vi "subSave_XYTfilename.vi"(4 "Xi":i32, 5 "Tiling?":bool, 6 "Yi":i32, 11 "Z-stack cluster in":T1={"Timelapse Acquired"=1, "File path"=path "C:/Users/ZouOptics/Desktop/TEST", "Z-Stack"={"Z end"=0.0, "Step Num"=1, "Step Size"=2.0, "Z0"=3471.0, "z-stack?"=FALSE}, "Frames to avg."=20, "Image Info Ref"=refnum, "Camera Ctrl"={"Chosen Camera"=0, "ROI selection"=0, "Live"=FALSE, "ROI define"=FALSE, "Snap"=FALSE, "ROI update"=FALSE, "ROI previous "=FALSE, "ROI"={"Bin"=2, "ROI"={"x offset"=256, "y offset"=256, "x width"=512, "y width"=512}}, "Exposure (ms)"=100.0, "Symmetrical"=FALSE, "Autoscale"=TRUE, "Scale"={"Scale.Min"=0, "Scale.Max"=6038}}} {"Camera Ctrl"."Scale"."Scale.Max" min=1 max=5000 step=1; "Camera Ctrl"."Scale"."Scale.Min" min=1 max=5000 step=1; "Camera Ctrl"."Exposure (ms)" min=1.0 max=5000.0 step=1.0; "Camera Ctrl"."ROI"."ROI"."x offset" min=1 max=512 step=1; "Camera Ctrl"."ROI"."ROI"."y offset" min=1 max=512 step=1; "Camera Ctrl"."ROI"."ROI"."x width" min=1 max=512 step=1; "Camera Ctrl"."ROI"."ROI"."y width" min=1 max=512 step=1; "Camera Ctrl"."ROI"."Bin" items=["1x1"=1, "2x2"=2, "4x4"=4]; "Camera Ctrl"."ROI selection" items=["Full ROI", "Central quad", "Confocal"]; "Camera Ctrl"."Chosen Camera" items=["Left", "Right"]}) -> (3 "Z-stack cluster out":T1={"Timelapse Acquired"=1, "File path"=path "C:/Users/ZouOptics/Desktop/TEST", "Z-Stack"={"Z end"=0.0, "Step Num"=1, "Step Size"=2.0, "Z0"=3471.0, "z-stack?"=FALSE}, "Frames to avg."=20, "Image Info Ref"=refnum, "Camera Ctrl"={"Chosen Camera"=0, "ROI selection"=0, "Live"=FALSE, "ROI define"=FALSE, "Snap"=FALSE, "ROI update"=FALSE, "ROI previous "=FALSE, "ROI"={"Bin"=2, "ROI"={"x offset"=256, "y offset"=256, "x width"=512, "y width"=512}}, "Exposure (ms)"=100.0, "Symmetrical"=FALSE, "Autoscale"=TRUE, "Scale"={"Scale.Min"=0, "Scale.Max"=6038}}} {"Camera Ctrl"."Scale"."Scale.Max" min=1 max=5000 step=1; "Camera Ctrl"."Scale"."Scale.Min" min=1 max=5000 step=1; "Camera Ctrl"."Exposure (ms)" min=1.0 max=5000.0 step=1.0; "Camera Ctrl"."ROI"."ROI"."x offset" min=1 max=512 step=1; "Camera Ctrl"."ROI"."ROI"."y offset" min=1 max=512 step=1; "Camera Ctrl"."ROI"."ROI"."x width" min=1 max=512 step=1; "Camera Ctrl"."ROI"."ROI"."y width" min=1 max=512 step=1; "Camera Ctrl"."ROI"."Bin" items=["1x1"=1, "2x2"=2, "4x4"=4]; "Camera Ctrl"."ROI selection" items=["Full ROI", "Central quad", "Confocal"]; "Camera Ctrl"."Chosen Camera" items=["Left", "Right"]})   [LabVIEW 2015]
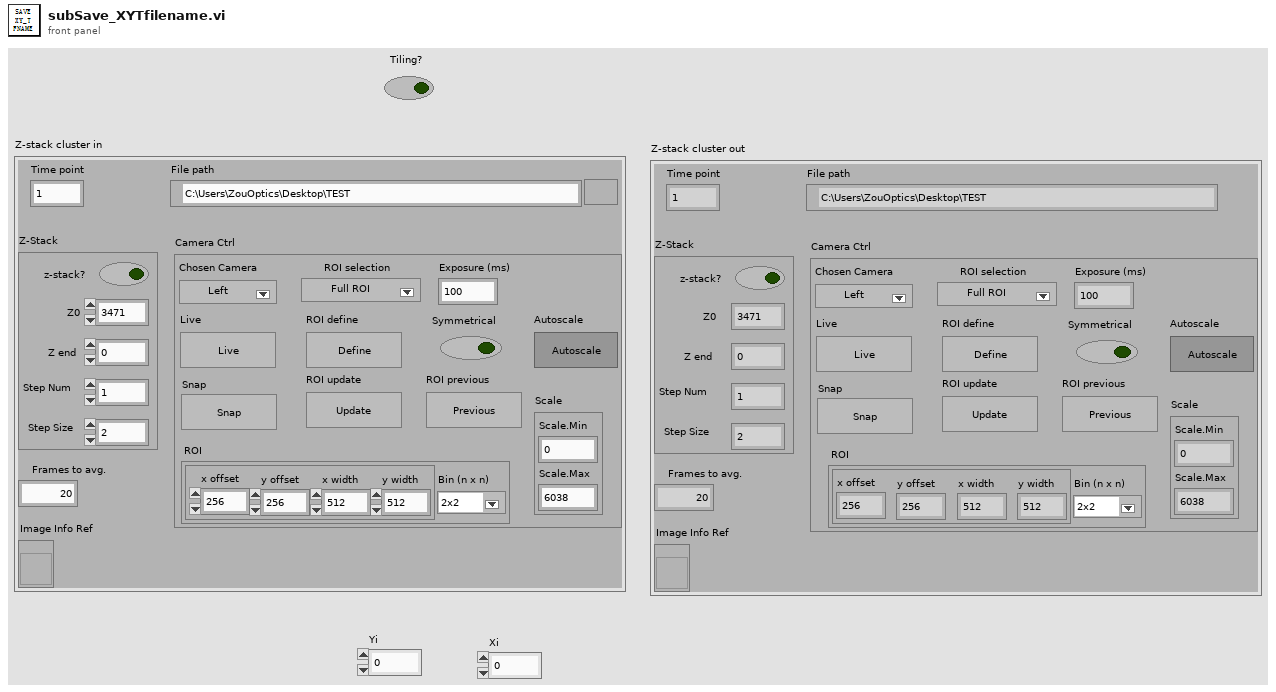
[diagram p1: front panel]
types:
  T1 = cluster{"Timelapse Acquired":i32, "File path":path, "Z-Stack":cluster{"Z end":dbl, "Step Num":i32, "Step Size":dbl, "Z0":dbl, "z-stack?":bool}, "Frames to avg.":i32, "Image Info Ref":refnum<vi>, "Camera Ctrl":cluster{"Chosen Camera":u32, "ROI selection":u16, "Live":bool, "ROI define":bool, "Snap":bool, "ROI update":bool, "ROI previous ":bool, "ROI":cluster{"Bin":u16, "ROI":cluster{"x offset":i32, "y offset":i32, "x width":i32, "y width":i32}}, "Exposure (ms)":dbl, "Symmetrical":bool, "Autoscale":bool, "Scale":cluster{"Scale.Min":i32, "Scale.Max":i32}}}
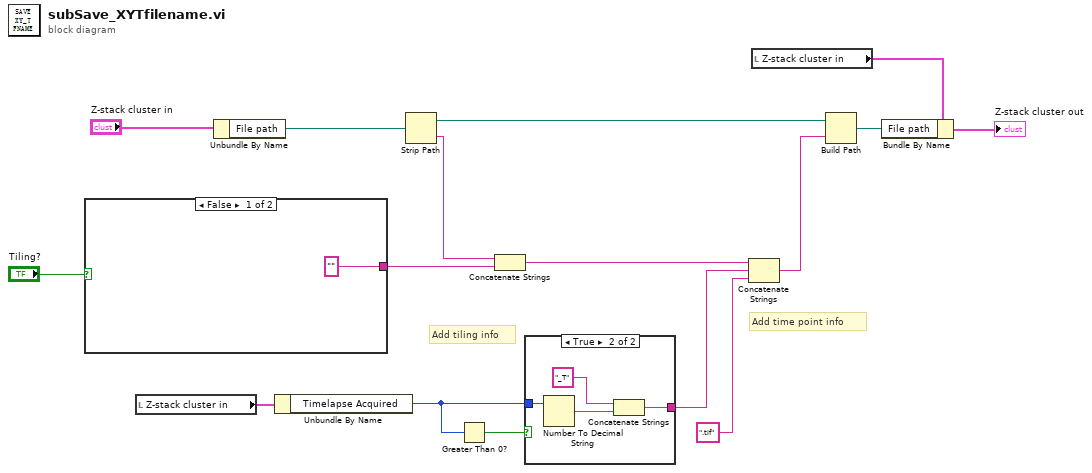
[diagram p0: block diagram]
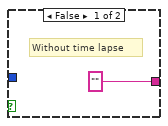
[diagram p2: hidden frame]
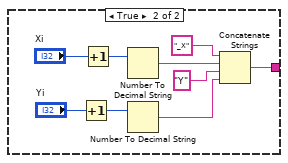
[diagram p3: hidden frame]
diagram:
  # "Add time point info"
  # "Add tiling info"
  n1 = case shown="False" "Tiling?" {
    tunnel: ["" w24] -> w10
    frame False {
    }
    frame True {
      n2 = Increment(x="Yi") -> (x+1=w25:i32)
      n3 = Increment(x="Xi") -> (x+1=w26:i32)
      n4 = Number To Decimal String(number=w26) -> (decimal integer string=w20:string)  [unwired: 1 in]
      n5 = Number To Decimal String(number=w25) -> (decimal integer string=w18:string)  [unwired: 1 in]
      n6 = Concatenate Strings("_X" ("string"), w20, "Y" ("string"), w18) -> (w24:string)
    }
  }
  n7 = local read "Z-stack cluster in"() -> (w13:T1)
  n8 = Unbundle By Name("Z-stack cluster in") -> ("File path"=w14:path)
  n9 = Unbundle By Name(w13) -> ("Timelapse Acquired"=w8:i32)
  n10 = Strip Path(path=w14) -> (stripped path=w16:path, name=w11:string)
  n11 = Greater Than 0?(x=w8) -> (x > 0?=w9:bool)
  n12 = Concatenate Strings(w11, w10) -> (w4:string)
  n13 = case shown="True" w9 {
    tunnel: w8 -> [_ w31]
    tunnel: ["" w28] -> w7
    frame False {
      # "Without time lapse"
    }
    frame True {
      n14 = Number To Decimal String(number=w31) -> (decimal integer string=w29:string)  [unwired: 1 in]
      n15 = Concatenate Strings("_T" ("string"), w29) -> (w28:string)
    }
  }
  n16 = Concatenate Strings(w4, w7, ".tif" ("string")) -> (w5:string)
  n17 = local read "Z-stack cluster in"() -> (w3:T1)
  n18 = Build Path(base path=w16, name or relative path=w5) -> (appended path=w2:path)
  n19 = Bundle By Name(cluster=w3, "File path"=w2) -> (→"Z-stack cluster out":T1)
